vi "Write Controller Data.vi"(10 "Controller Data":T1 {"Force Error" min=-888.0 max=888.0 format="%.2f"; "Force Setpoint" min=-888.0 max=888.0 format="%.2f"}, 11 "Logger in":refnum<class "TestDataLog.lvclass">) -> (3 "Logger out":refnum<class "TestDataLog.lvclass">)   [LabVIEW 2013, in "TestDataLog.lvclass"]
uses:
  TestDataLog.lvclass
  Typedefs/ControllerData.ctl
  Typedefs/ForceSetpoint.ctl
  TestDataLog.lvclass/TestDataLog.ctl
  Typedefs/FAMTTypedefs.lvlib
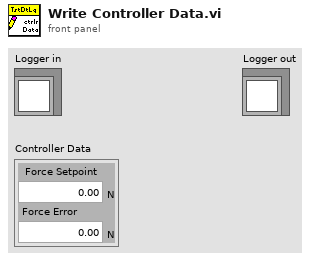
[diagram p1: front panel]
types:
  T1 = typedef "FAMTTypedefs.lvlib/ControllerData.ctl" = cluster{"Force Setpoint":T2, "Force Error":T2}
  T2 = typedef "FAMTTypedefs.lvlib/ForceSetpoint.ctl" = dbl[unit]
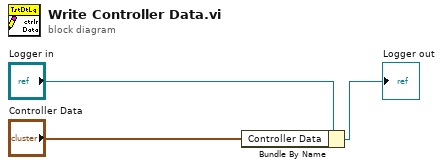
[diagram p0: block diagram]
diagram:
  n1 = Bundle By Name(cluster="Logger in", "Controller Data"="Controller Data") -> (→"Logger out":refnum<class "TestDataLog.lvclass">)
